vi "rsscope_FormatLabelSourceBoolean_ReadCallback.vi"(5 "Attribute":T1={"Identifier"="", "Descriptive Name"="", "Data Type"=enum."Integer 32", "Command"="", "Access"=enum."Read/Write", "Range Table"="", "Read Callback"="", "Write Callback"="", "Supported Models"="", "Instrument Options"="", "Index"=0, "OPC Wait"=FALSE, "No Status Check"=FALSE, "Cache Only"=FALSE}, 7 "Repeated Capability":string, 8 "error in (no error)":errorcluster, 11 "VISA resource name":refnum<visa-resource-name>) -> (0 "error out":errorcluster, 2 "Attribute Value Boolean":bool, 3 "VISA resource name out":refnum<visa-resource-name>)   [LabVIEW 2018]
doc: "This VI sets the attribute value.\n\nThis is a low-level VI that you can use to set the values of instrument-specific properties and inherent IVI properties. If the property represents an instrument state, this VI performs instrument I/O in the following cases:\n\n- State caching is disabled for the entire session or for the particular property.\n\n- State caching is enabled and the currently cached value is invalid or is different than the value you specify. \n\nThis instrument driver contains high-level VIs that set most of the instrument properties. It is best to use the high-level driver VIs as much as possible. They handle order dependencies and multithread locking for you. In addition, they perform status checking only after setting all of the properties. In contrast, when you set multiple properties using the SetAttribute VIs, the VIs check the instrument status after each call.\n\nAlso, when state caching is enabled, the high-level VIs that configure multiple properties perform instrument I/O only for the properties whose value you change. Thus, you can safely call the high-level VIs without the penalty of redundant instrument I/O."
uses:
  rsidr_core.llb/type_Attribute.ctl
  rsidr_core.llb/type_Attribute_Data_Type.ctl
  rsidr_core.llb/type_ReadWriteAccess.ctl
  rsidr_core.llb/rsscope_rsidr_core.lvlib
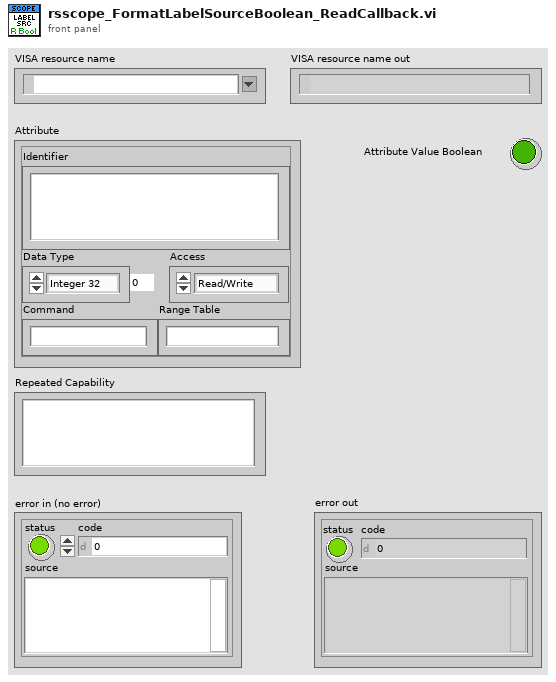
[diagram p1: front panel]
types:
  T1 = typedef "rsscope_rsidr_core.lvlib/type_Attribute.ctl" = cluster{"Identifier":string, "Descriptive Name":string, "Data Type":T2, "Command":string, "Access":T3, "Range Table":string, "Read Callback":string, "Write Callback":string, "Supported Models":string, "Instrument Options":string, "Index":i32, "OPC Wait":bool, "No Status Check":bool, "Cache Only":bool}
  T2 = typedef "rsscope_rsidr_core.lvlib/type_Attribute_Data_Type.ctl" = enum16{"Integer 32", "Double", "String", "Boolean", "None", "Integer 64", "RawString"}
  T3 = typedef "rsscope_rsidr_core.lvlib/type_ReadWriteAccess.ctl" = enum16{"Read Only", "Write Only", "Read/Write"}
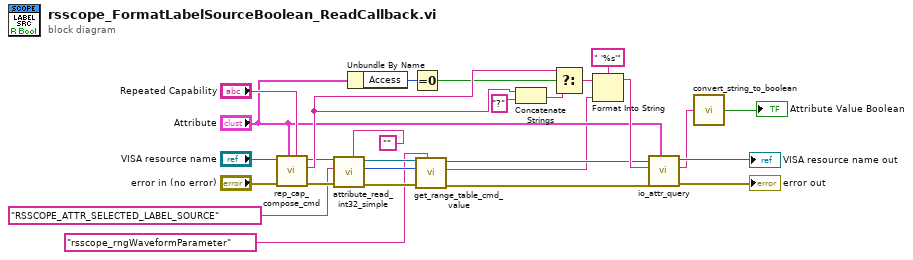
[diagram p0: block diagram]
diagram:
  n1 = call "rep_cap_compose_cmd.vi"("Repeated Capability"="Repeated Capability", "Attribute"="Attribute", "error in"="error in (no error)", "VISA resource name"="VISA resource name") -> ("error out"=w10:errorcluster, "Command out"=w22:string, "VISA resource name out"=w11:refnum<visa-resource-name>)  [unwired: 5 in]
  n2 = call "attribute_read_int32_simple.vi"("Repeated Capability"="" ("Empty String Constant"), "error in"=w10, "Direct Attribute ID (\"\")"="RSSCOPE_ATTR_SELECTED_LABEL_SOURCE" ("Direct Attribute ID (\"\")"), "VISA resource name"=w11) -> ("error out"=w6:errorcluster, "Int32 out"=w5:i32, "VISA resource name out"=w7:refnum<visa-resource-name>)  [unwired: 5 in]
  n3 = Unbundle By Name("Attribute") -> ("Access"=w19:T3)
  n4 = Equal To 0?(x=w19) -> (x = 0?=w18:bool)
  n5 = call "get_range_table_cmd_value.vi"("Range Table ID in"="rsscope_rngWaveformParameter", "error in"=w6, "Input Int32 value"=w5, "VISA resource name"=w7) -> ("error out"=w2:errorcluster, "Cmd value out"=w1:string, "VISA resource name out"=w3:refnum<visa-resource-name>)  [unwired: 5 in]
  n6 = Concatenate Strings(w22, "?" ("string")) -> (w21:string)
  n7 = Select(t=w22, s=w18, f=w21) -> (s? t:f=w17:string)
  n8 = Format Into String(format string=" '%s'", initial string=w17, w1) -> (resulting string=w16:string)  [unwired: 1 in, 1 out]
  n9 = call "io_attr_query.vi"("Attribute"="Attribute", "error in"=w2, "write buffer"=w16, "VISA resource name"=w3) -> ("error out"=→"error out":errorcluster, "read buffer"=w13:string, "VISA resource name out"=→"VISA resource name out":refnum<visa-resource-name>)  [unwired: 5 in]
  n10 = call "convert_string_to_boolean.vi"("String in"=w13) -> ("boolean value out"=→"Attribute Value Boolean":bool)  [unwired: 4 in]
